vi "MPU6050 Read Z Rotation.vi"(8 "error in (no error)":errorcluster, 10 "Gyro Bias":dbl, 11 "I2C Ref In":T1={"myRIO Reference"={"myRIO Model"=enum."Unknown", "myRIO Hardware Reference"={"Generic FPGA Reference"=refnum, "Allow multiple opens"=FALSE}}, "I2C Channels Enum"=enum."Not Connected", "I2C Configuration"={"I2C Transfer Rate"=enum."Fast mode (400 kbps)"}}) -> (0 "error out":errorcluster, 3 "Z Rotation (rads)":dbl)   [LabVIEW 2017]
uses:
  <vilib>/myRIO/Instrument Drivers/Onboard IO/I2C/typedefs/I2C Reference.ctl
  <vilib>/myRIO/Common/Instrument Driver Framework/Utilities/typedefs/myRIO Generic Hardware Reference.ctl
  <vilib>/myRIO/Common/Instrument Driver Framework/Utilities/typedefs/Hardware Version Enum.ctl
  <vilib>/myRIO/Common/Instrument Driver Framework/Utilities/typedefs/myRIO v1.0 Reference.ctl
  <vilib>/myRIO/Common/Instrument Driver Framework/Utilities/typedefs/Generic FPGA Reference.ctl
  <vilib>/myRIO/Common/Instrument Driver Framework/myRIO v1.0/I2C/typedefs/I2C Channels Enum.ctl
  <vilib>/myRIO/Instrument Drivers/Onboard IO/I2C/typedefs/I2C Configuration.ctl
  <vilib>/myRIO/Instrument Drivers/Onboard IO/I2C/typedefs/I2C Transfer Rate.ctl
  <vilib>/myRIO/Instrument Drivers/Onboard IO/I2C/I2C.lvlib
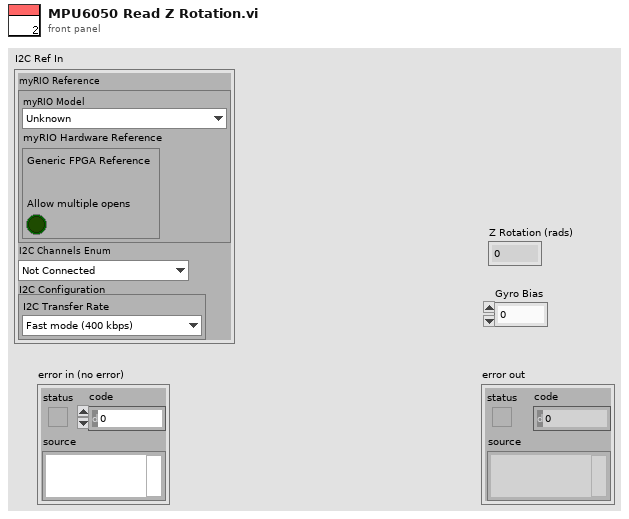
[diagram p1: front panel]
types:
  T1 = typedef "I2C.lvlib/I2C Reference.ctl" = cluster{"myRIO Reference":T2, "I2C Channels Enum":T6, "I2C Configuration":T7}
  T2 = typedef "myRIO Generic Hardware Reference.ctl" = cluster{"myRIO Model":T3, "myRIO Hardware Reference":T4}
  T3 = typedef "Hardware Version Enum.ctl" = enum16{"Unknown", "myRIO-1900", "myRIO-1950", "roboRIO", "NI ELVIS RIO CM"}
  T4 = typedef "myRIO v1.0 Reference.ctl" = cluster{"Generic FPGA Reference":T5, "Allow multiple opens":bool}
  T5 = typedef "Generic FPGA Reference.ctl" = refnum<k20>
  T6 = typedef "I2C Channels Enum.ctl" = enum16{"Not Connected", "A/I2C", "B/I2C", "I2C/I2C"}
  T7 = typedef "I2C.lvlib/I2C Configuration.ctl" = cluster{"I2C Transfer Rate":T8}
  T8 = typedef "I2C.lvlib/I2C Transfer Rate.ctl" = enum16{"Standard mode (100 kbps)", "Fast mode (400 kbps)"}
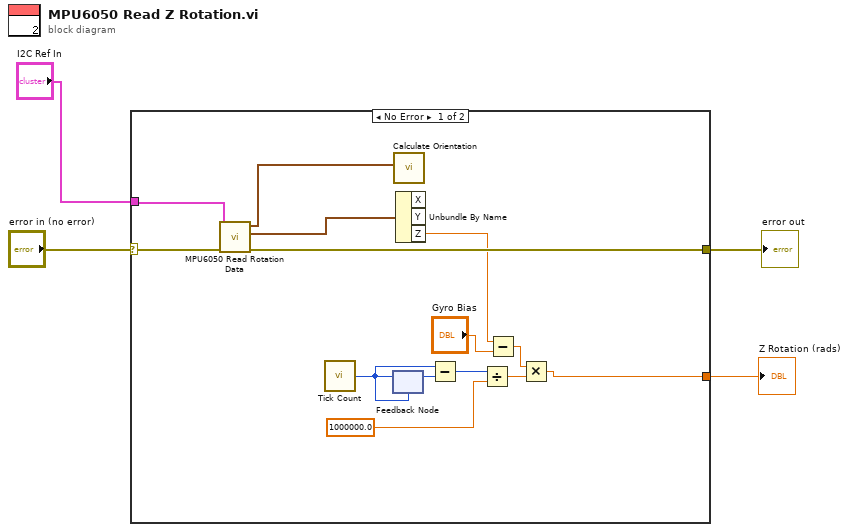
[diagram p0: block diagram]
diagram:
  n1 = case shown="No Error" "error in (no error)" {
    selector: "error in (no error)" -> [w18 w19]
    tunnel: [w17 w19] -> w4
    tunnel: [w7 _] -> w3
    tunnel: "I2C Ref In" -> [w10 _]
    frame No Error {
      n2 = call "MPU6050 Read Rotation Data.vi"("error in (no error)"=w18, "I2C Ref In"=w10) -> ("error out"=w17:errorcluster, "rad/s"=w14:cluster{"X":dbl, "Y":dbl, "Z":dbl}, "Accel"=w5:cluster{dbl, dbl, dbl})  [unwired: 7 in]
      n3 = call "Tick Count"() -> ("Tick Count(uSec)"=w16:u32)
      n4 = feedback-in #1(w16) -> ()
      n5 = feedback #1(w16) -> (w15:u32)
      n6 = call "Calculate Orientation.vi"("Accel"=w5) -> ()  [unwired: 11 in]
      n7 = Unbundle By Name(w14) -> ("Z"=w6:dbl)  [unwired: 2 out]
      n8 = Subtract(x=w16, y=w15) -> (x-y=w13:u32)
      n9 = Divide(x=w13, y=1000000.0) -> (x/y=w11:dbl)
      n10 = Subtract(x=w6, y="Gyro Bias") -> (x-y=w8:dbl)
      n11 = Multiply(x=w8, y=w11) -> (x*y=w7:dbl)
    }
    frame Error {
    }
  }
  "error out" <- w4
  "Z Rotation (rads)" <- w3
